vi "RT Main.vi"() -> ()   [LabVIEW 2017]
uses:
  Vibration.ctl
  <vilib>/DAQmx/read.llb/DAQmx Read (Analog Wfm 1Chan NSamp).vi
  <extravilib>/ChannelInstances/Stream-t'Vibration.ctl'/Read With Abort.vi
  <extravilib>/ChannelInstances/Stream-wfm(dbl)/Read With Abort.vi
  <extravilib>/ChannelInstances/Stream-t'Vibration.ctl'/Write With Abort.vi
  <extravilib>/ChannelInstances/Stream-t'Vibration.ctl'/EndpointRead.vi
  <extravilib>/ChannelInstances/Stream-wfm(dbl)/EndpointRead.vi
  <extravilib>/ChannelInstances/Stream-t'Vibration.ctl'/Endpoint.vi
  <vilib>/DAQmx/create/channels.llb/DAQmx Create Channel (AI-Voltage-Basic).vi
  <vilib>/DAQmx/configure/timing.llb/DAQmx Timing (Sample Clock).vi
  <extravilib>/ChannelInstances/Stream-wfm(dbl)/Instantiate.vi
  <extravilib>/ChannelInstances/Stream-wfm(dbl)/)Channel.vi
  <resource>/ChannelSupport/_ChannelSupport/WaitIfNeeded.vi
  <vilib>/Skyline/File/File/Send File.vi
  <extravilib>/ChannelInstances/Stream-t'Vibration.ctl'/Instantiate.vi
  <extravilib>/ChannelInstances/Stream-t'Vibration.ctl'/)Channel.vi
  <vilib>/DAQmx/miscellaneous.llb/DAQmx Fill In Error Info.vi
  <extravilib>/ChannelInstances/Stream-t'Vibration.ctl'.lvlib
  <vilib>/Skyline/File/File/NI Skyline File.lvclass
  <extravilib>/ChannelInstances/Stream-wfm(dbl).lvlib
panel:
  in  "Measure Time (s)":dbl
  out "RMS":dbl=nan format="%.6f"
  in  "Vibration Sample":i32=51200
  in  "Chamber Name":string
  in  "Max-Min Threshold":dbl
  out "Max-Min":dbl=nan format="%.6f"
  out "Vibration Alarm":bool
  in  "RMS Threshold":dbl
  in  "Intervals (s)":dbl=1.0 caption="Time Target (s)"
  in  "Stop Button":bool
  out "Vibration":waveform(dbl)(graph)
  in  "Vibration Sample Rate":dbl=51200.0
  in  "Vibration  Channel":tag="Mod1/ai0"
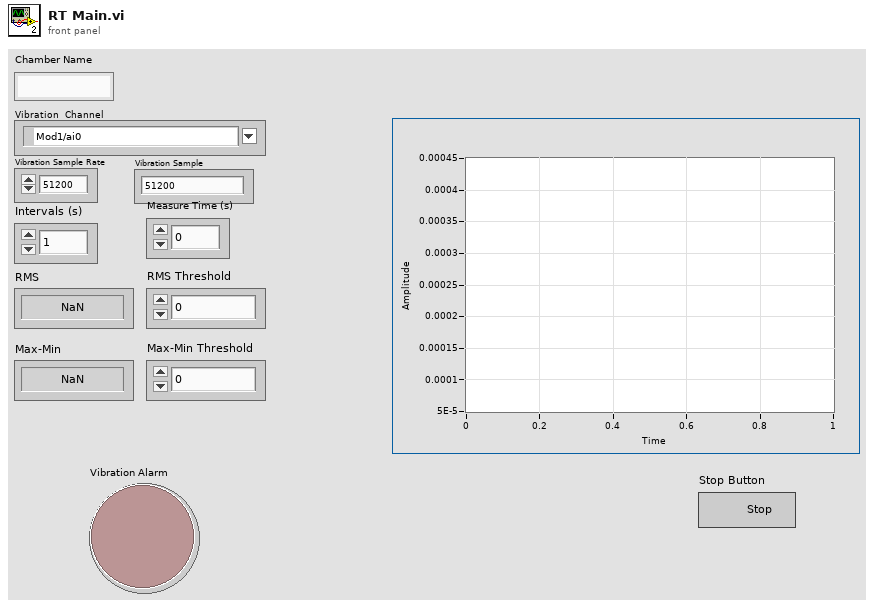
[diagram p1: front panel]
types:
  T1 = cluster{"Count":i32, "Total Count":dbl, "data":waveform(dbl)}
  T2 = typedef "Vibration.ctl" = cluster{"Vibration Wfm Data":waveform(dbl), "RMS":dbl, "Max-Min":dbl, "RMS Alarm":bool, "Max-Min Alarm":bool, "Vibration Alarm":bool, "Chamber Name":string}
  T3 = typedef "Stream-t'Vibration.ctl'.lvlib/)Channel.ctl" = refnum<queue>
  T4 = typedef "Stream-wfm(dbl).lvlib/)Channel.ctl" = refnum<queue>
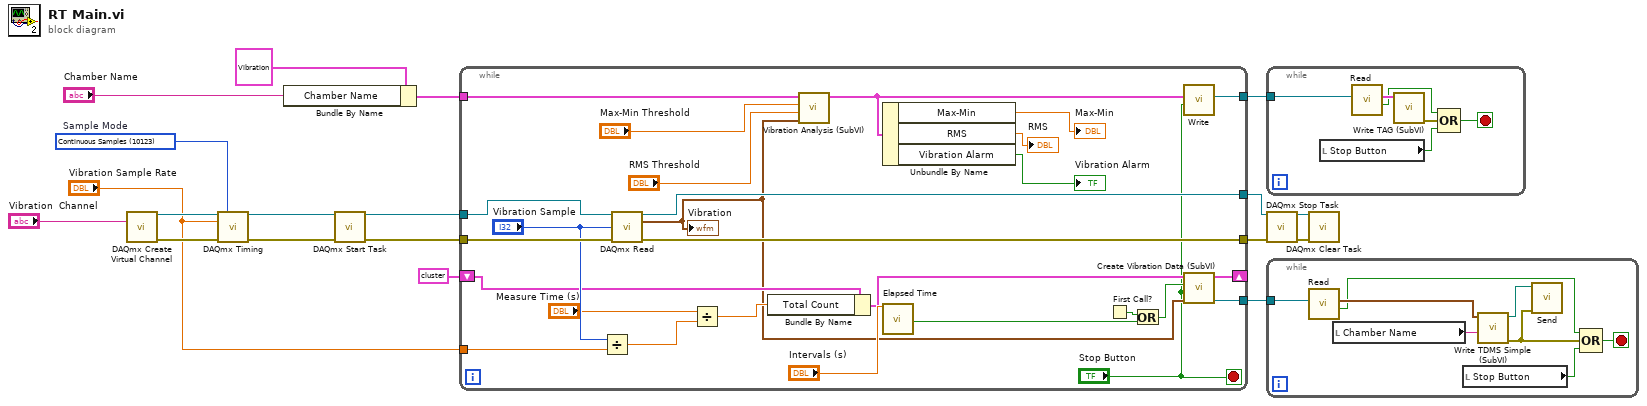
[diagram p0: block diagram]
diagram:
  w11 = 10123 items=["Finite Samples"=10178, "Continuous Samples"=10123, "Hardware Timed Single Point"=12522]  # Sample Mode
  n1 = call-poly <vilib>:"DAQmx Create Virtual Channel.vi"("physical channels"="Vibration  Channel") -> ("task out"=w15:refnum<k21>, "error out"=w14:errorcluster)  [unwired: 13 in]
  n2 = call-poly <vilib>:"DAQmx Timing.vi"("task/channels in"=w15, "sample mode"=w11, "rate"="Vibration Sample Rate", "error in"=w14) -> ("task out"=w12:refnum<k21>, "error out"=w13:errorcluster)  [unwired: 10 in]
  n3 = Bundle By Name(cluster=T2 {"Vibration Wfm Data"={"t0"=timestamp(3614627182.308542 s since 1904-01-01), "dt"=0.0, "Y"=array[51200 elements], "attributes"=variant("NI_ChannelName"=variant(string "Mod1/ai0"), "NI_UnitDescription"=variant(string "Volts"))}, "RMS"=0.0, "Max-Min"=0.0, "RMS Alarm"=FALSE, "Max-Min Alarm"=FALSE, "Vibration Alarm"=FALSE, "Chamber Name"=""} ("Cluster"), "Chamber Name"="Chamber Name") -> (w18:T2)
  n4 = call <vilib>:"DAQmx Start Task.vi"("task/channels in"=w12, "error in"=w13) -> ("task out"=w10:refnum<k21>, "error out"=w9:errorcluster)  [unwired: 12 in]
  n5 = while {
    tunnel: w18 -> [w41]
    tunnel: w10 -> [w45]
    tunnel: w9 -> [w44]
    tunnel: [w43] -> w6
    tunnel: [w42] -> w5
    tunnel: "Vibration Sample Rate" -> [w35]
    shift-right: [w25] -> _
    shift-left: T1 {"Count"=0, "Total Count"=0.0, "data"={"t0"=timestamp(0 s since 1904-01-01), "dt"=0.0, "Y"=[]}} -> [w30]
    tunnel: [w24] -> w1
    tunnel: [w28] -> w2
    stop <- "Stop Button" stop-if-true
    n6 = Divide(x="Vibration Sample", y=w35) -> (x/y=w33:dbl)
    n7 = call-poly <vilib>:"DAQmx Read.vi"("task/channels in"=w45, "number of samples per channel"="Vibration Sample", "error in"=w44) -> ("task out"=w43:refnum<k21>, "data"=w26:waveform(dbl), "error out"=w42:errorcluster)  [unwired: 10 in]
    "Vibration" <- w26
    n8 = Divide(x="Measure Time (s)", y=w33) -> (x/y=w31:dbl)
    n9 = Bundle By Name(cluster=w30, "Total Count"=w31) -> (w27:T1)
    n10 = call "Vibration Analysis (SubVI).vi"("data"=w26, "RMS Threshold"="RMS Threshold", "Max-Min Threshold"="Max-Min Threshold", "Cluster"=w41) -> ("output cluster"=w29:T2)  [unwired: 7 in]
    n11 = Unbundle By Name(w29) -> ("Max-Min"=→"Max-Min":dbl, "RMS"=→"RMS":dbl, "Vibration Alarm"=→"Vibration Alarm":bool)
    n12 = call "Elapsed Time"("Time Target (s)"="Intervals (s)") -> ("Time has Elapsed"=w22:bool)  [unwired: 11 in, 7 out]
    n13 = First Call?() -> (First Call?: T/F=w21:bool)
    n14 = Or(x=w21, y=w22) -> (x .or. y?=w23:bool)
    n15 = call <extravilib>:"Write.vi"("last element? (F)"="Stop Button", "element"=w29) -> ("channel"=w28:T3)  [unwired: 7 in, 2 out]
    n16 = call "Create Vibration Data (SubVI).vi"("data"=w26, "Stop"="Stop Button", "Time has Elapsed"=w23, "Cluster in"=w27) -> ("Channel out"=w24:T4, "Cluster out"=w25:T1)  [unwired: 5 in]
  }
  n17 = while {
    tunnel: w2 -> [w52]
    stop <- w50 stop-if-true
    n18 = local read "Stop Button"() -> (w48:bool)
    n19 = call <extravilib>:"Read.vi"("channel"=w52) -> ("last element?"=w47:bool, "element"=w51:T2)  [unwired: 6 in, 3 out]
    n20 = call "Write TAG (SubVI).vi"("element"=w51) -> ("error out"=w49:errorcluster)  [unwired: 10 in]
    n21 = Compound Arithmetic op=OR(w47, w49, w48) -> (w50:bool)
  }
  n22 = call <vilib>:"DAQmx Stop Task.vi"("task/channels in"=w6, "error in"=w5) -> ("task out"=w7:refnum<k21>, "error out"=w8:errorcluster)  [unwired: 12 in]
  n23 = while {
    tunnel: w1 -> [w60]
    stop <- w56 stop-if-true
    n24 = call <extravilib>:"Read.vi"("channel"=w60) -> ("last element?"=w53:bool, "element"=w58:waveform(dbl))  [unwired: 6 in, 3 out]
    n25 = local read "Chamber Name"() -> (w57:string)
    n26 = local read "Stop Button"() -> (w54:bool)
    n27 = call "Write TDMS Simple (SubVI).vi"("string"=w57, "element"=w58) -> ("error out"=w55:errorcluster, "file path out"=w59:path)  [unwired: 8 in]
    n28 = call-poly <vilib>:"Send.vi"("error in (no error)"=w55, "path"=w59) -> ()  [unwired: 7 in, 2 out]
    n29 = Compound Arithmetic op=OR(w53, w55, w54) -> (w56:bool)
  }
  n30 = call <vilib>:"DAQmx Clear Task.vi"("task in"=w7, "error in"=w8) -> ()  [unwired: 13 in, 1 out]
